vi "play_AFMss_integral_trajTrack_nod.vi"() -> ()   [LabVIEW 2017]
uses:
  controls/controlParams_tracktraj.ctl
  <vilib>/userdefined/High Color/nirio_resource_hc.ctl
  <vilib>/Utility/file.llb/Read From Spreadsheet File (DBL).vi
  <vilib>/FPGAPlugInAG/cRIO-9082/niLvFpga_Open_cRIO-9082.vi
  <vilib>/rvi/interface/common/dynamic/niFpgaDynamicAddResources.vi
  <vilib>/FPGAPlugInAG/Dynamic/niLvFpga_Reset_Dynamic.vi
  <vilib>/rvi/interface/common/niFpgaWaitOnOcc.vi
  <vilib>/Utility/error.llb/Error Cluster From Error Code.vi
  <vilib>/rvi/errors/niLvFpgaAdjustHostInterfaceError.vi
  <vilib>/FPGAPlugInAG/Dynamic/niLvFpga_Run_Dynamic.vi
  <vilib>/Utility/file.llb/Write To Spreadsheet File (DBL).vi
  <vilib>/FPGAPlugInAG/Dynamic/niLvFpga_Close_Dynamic.vi
  <vilib>/rvi/interface/nirviOpenFPGA/nirviOpenFPGA.xnode
  FPGA Bitfiles/XYpeizocontrol_FPGATargetSPARTA_AFMsscontroltraj_COTITsTKvb4.lvbitx
  <vilib>/rvi/interface/nirviMethod/nirviMethod.xnode
  <vilib>/rvi/interface/nirviReadWriteControl/nirviReadWriteControl.xnode
  <vilib>/rvi/interface/nirviCloseFPGA/nirviCloseFPGA.xnode
  <vilib>/FPGAPlugInAG/Dynamic/niLvFpga_ConfigureFifo_Dynamic.vi
  <vilib>/rvi/errors/niLvFpgaMergeErrorWithErrorCode.vi
  <vilib>/rvi/interface/Simulation/niFpgaSimulationCallBeginRW.vi
  <vilib>/FPGAPlugInAG/Dynamic/niLvFpga_ReadFifo_Dynamic.vi
  <vilib>/FPGAPlugInAG/Dynamic/niLvFpga_WriteFifo_Dynamic.vi
  NiFpgaLv.dll
panel:
  out "output array":dbl[][](array[numeric])
  in  "control_data_path":path=path "Z:/mpc-journal/step-exps/exp01Controls.csv"
  out "Actual Depth":u32
  out "YK TO":bool
  out "UK TO":bool
  out "yk":sgl
  out "loop ticks benchmark":sgl
  in  "Cluster":T1={"umax"=3.0, "y_ref(k)"=0.0, "Ki"=0.0, "y(k) (from plant)"=0.0, "ND"=0, "NS"=0, "u_Kx_ref(k)"=0.0} {"u_Kx_ref(k)" format="%#_13g"; "Ki" format="%#_13g"; "y_ref(k)" format="%#_13g"; "umax" format="%#_13g"}
  out "Unstable Traj":bool
  out "Control Loop Done":bool
  out "Elements Remaining":u32
  out "elements left":i32=1
  in  "reference traj path":path=path "Z:/mpc-journal/step-exps/ref_traj_track.csv"
  in  "outputData BOTH":path=path "Z:/mpc-journal/step-exps/exp01outputBOTH.csv"
  out "x+1":i32
  out "ND":i32
  out "NS":i32
  in  "Tab Control":enum32{"Custom Params", "Loaded Params"}(tab)
  in  "Nbar":dbl=1.253469179440319 format="%#_13g"
  in  "Ki":dbl=0.125346917944 format="%#_13g"
  out "Nbar":dbl=1.253469179440319 format="%#_13g"
  out "Ki":dbl=0.125346917944 format="%#_13g"
  out "ref":dbl format="%#_13g"
  in  "SettleTicks":i32=10
  in  "Stop":bool=TRUE
  out "y iter":i32
  out "u iter":i32
  out "size(s) 5":i32
  out "size(s)":i32
  out "K_in 2":sgl[](array[numeric])=[-0.023819132, 0.00010408472, 0.0, 0.0, 0.0, 0.0, 0.0, 0.0, 0.0]
  out "K_in":sgl[](array[numeric])=[-0.023819132, 0.00010408472, 0.0, 0.0, 0.0, 0.0, 0.0, 0.0, 0.0]
  out "C_in":sgl[](array[numeric])=[-8.076578e-08, -5.6617e-09, 2.3556278e-05, -6.9169624e-07, -0.005420799, 0.00037984832, -0.012524399, 0.0, 0.0]
  out "L_in":sgl[](array[numeric])=[-2254.4756, -17288.861, -3886.0125, -24956.67, -705.887, -3987.6506, -7.2153935, 0.0, 0.0] format="%#_11g"
  out "Bz_in":sgl[](array[numeric])=[-0.0016434871, -0.020676594, -0.010679029, -0.20639984, -0.030792456, -1.3413852, -0.02736353, 0.0, 0.0]
  in  "Iters":i32=25
  in  "Cont Run (F)":bool=TRUE
  in  "ymax":dbl=4.0 format="%#_13g"
  in  "umax":dbl=1.0 format="%#_13g"
  in  "TsTicks":i32=1600
  # "Manually define Parameters"
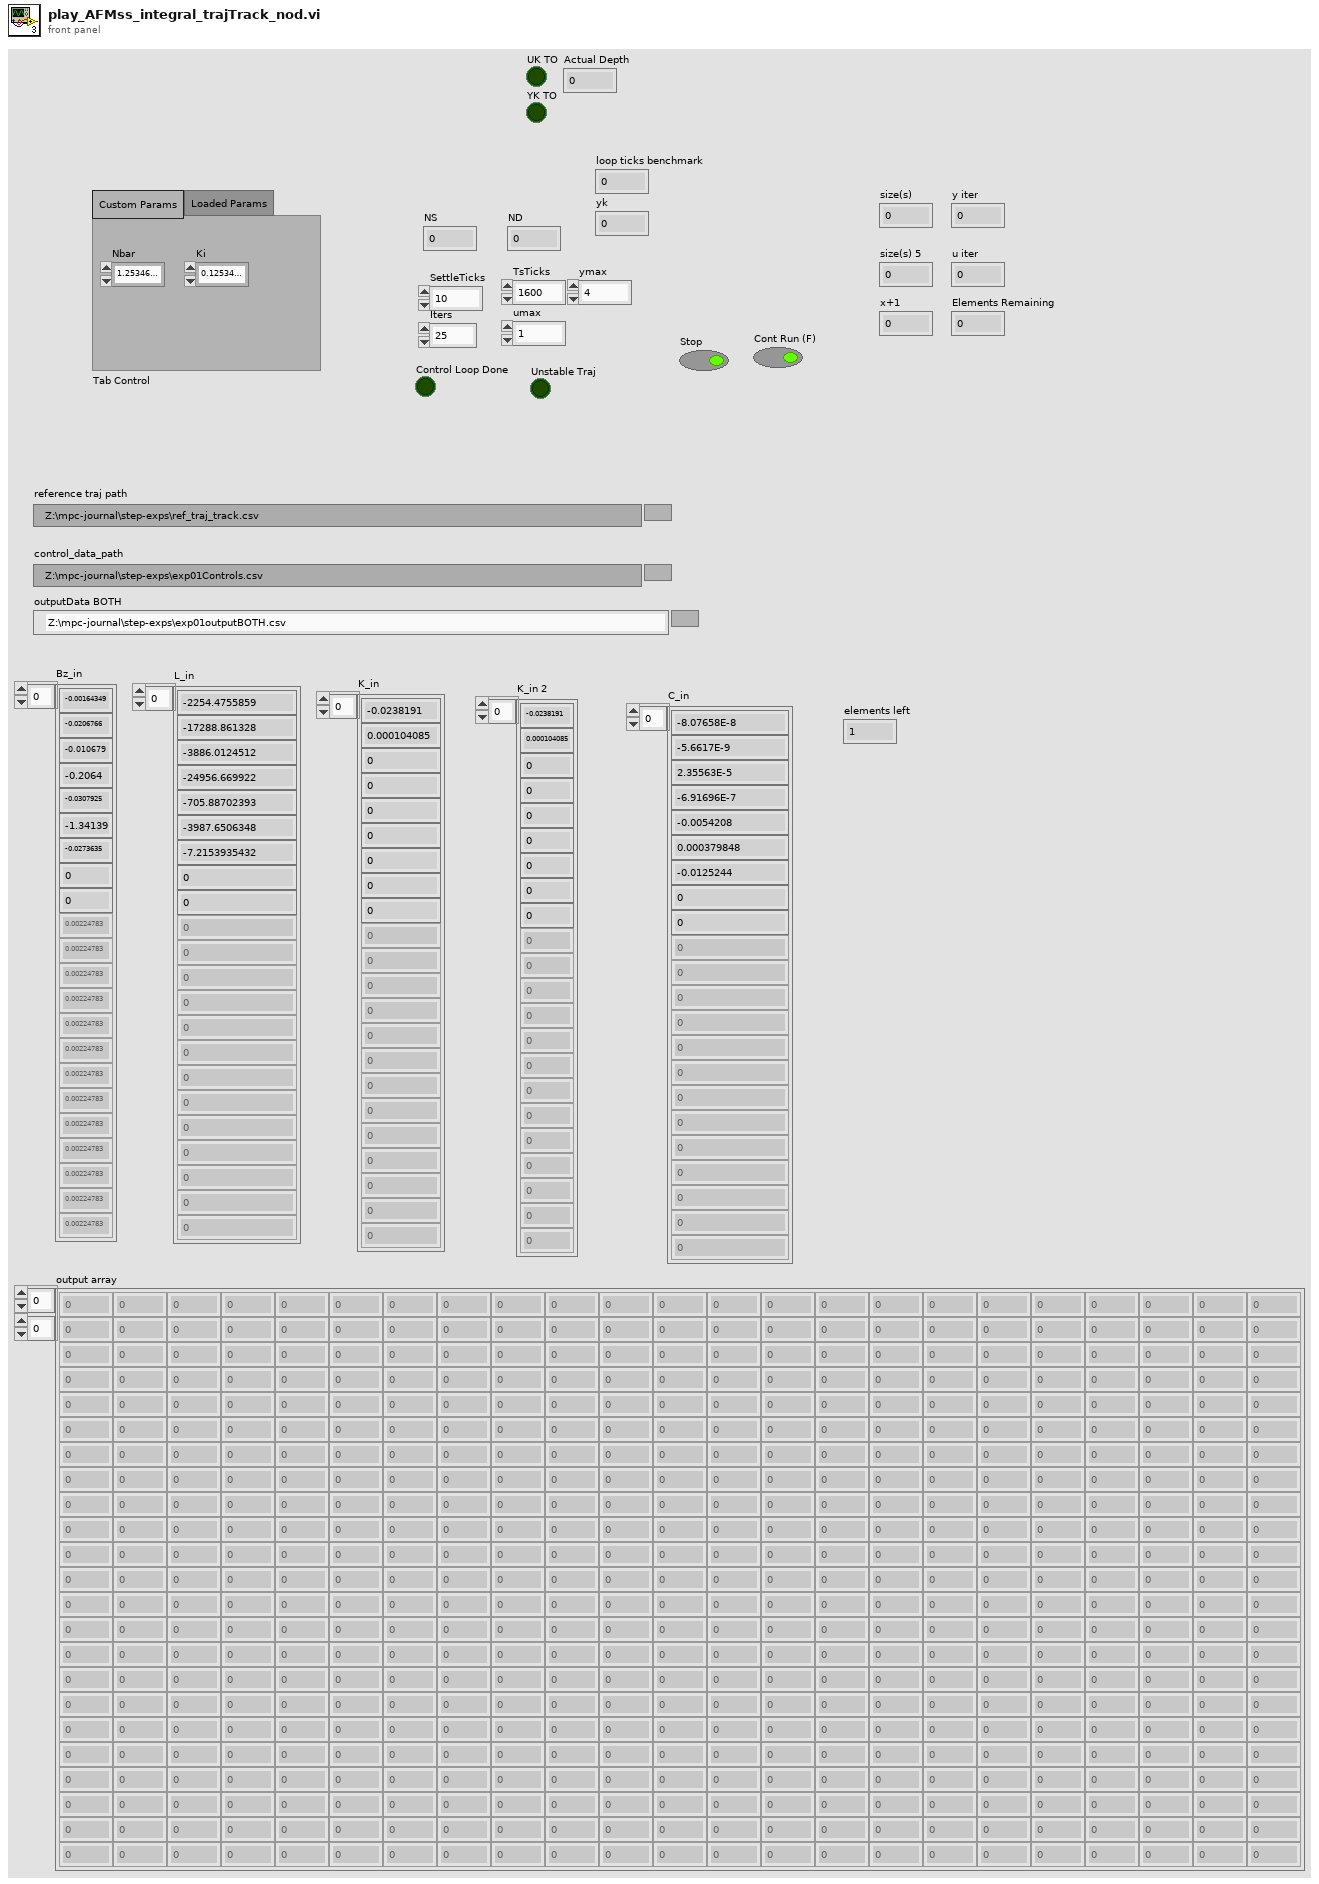
[diagram p1: front panel]
types:
  T1 = typedef "controlParams_tracktraj.ctl" = cluster{"umax":sgl, "y_ref(k)":sgl, "Ki":sgl, "y(k) (from plant)":sgl, "ND":i16, "NS":i16, "u_Kx_ref(k)":sgl}
  T2 = typedef "nirio_resource_hc.ctl" = tag
  T3 = typedef "ControlParams.ctl" = cluster{"NS":i32, "ND":i32, "Nbar":dbl, "Ki":dbl, "ref":dbl}
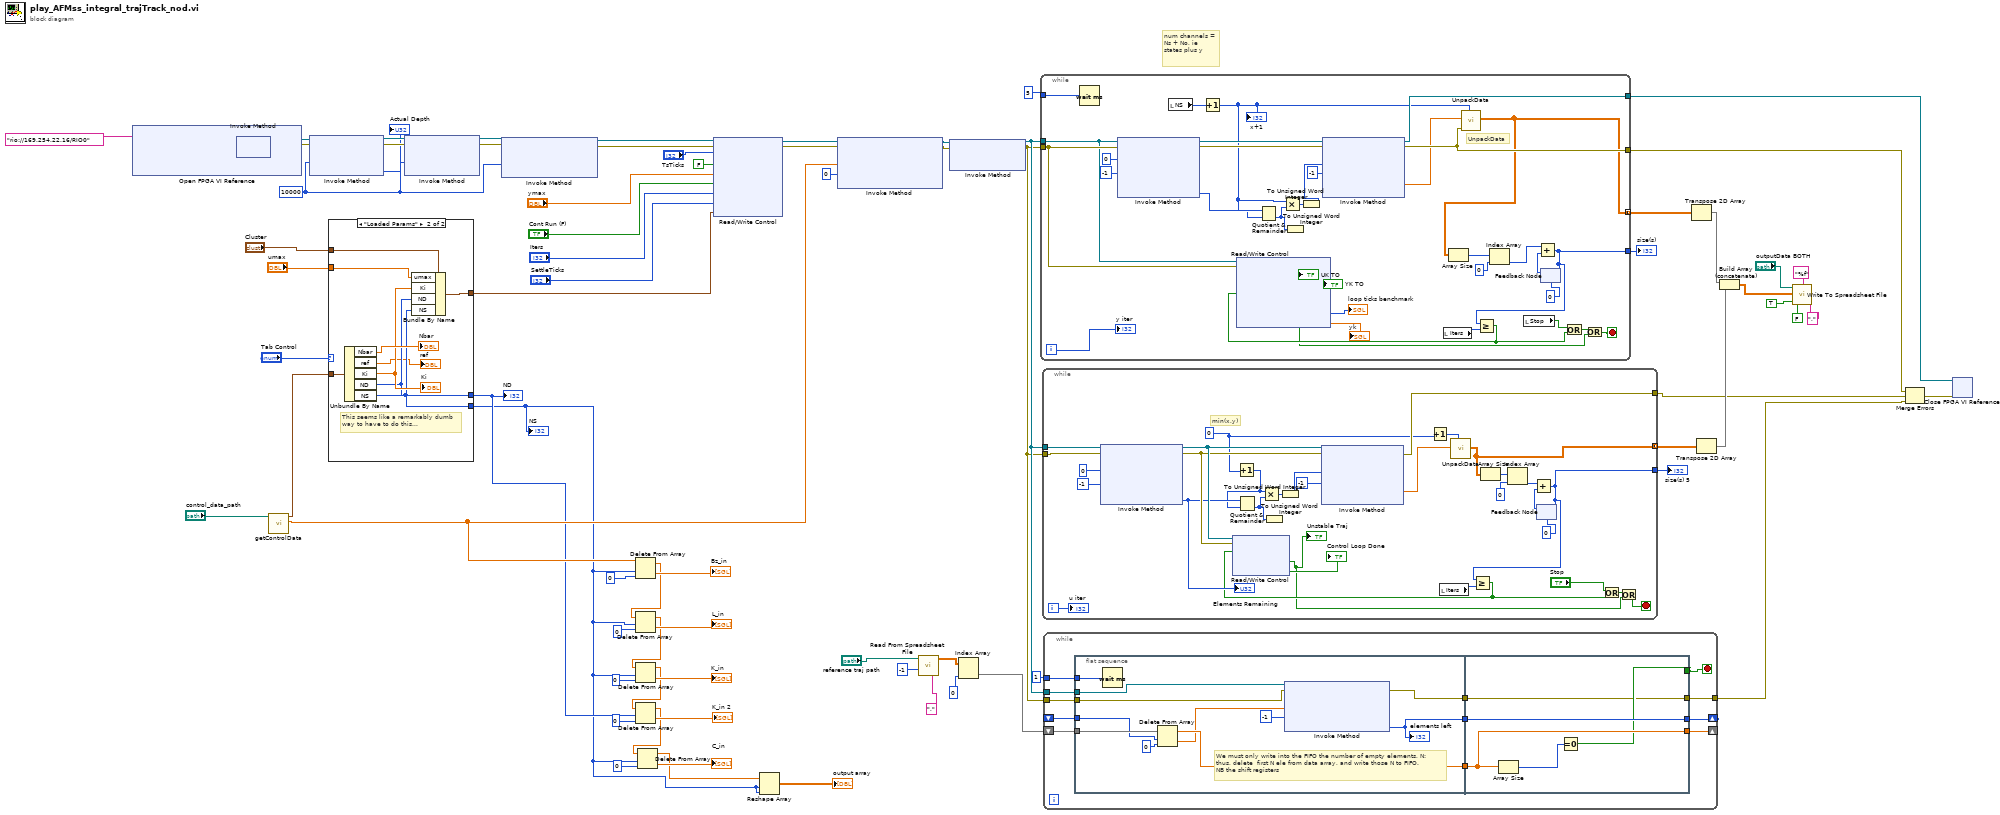
[diagram p0: block diagram]
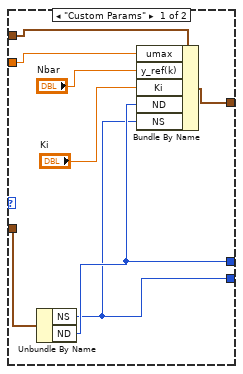
[diagram p2: hidden frame]
diagram:
  w38 = 10000
  # "num channels = Ns + No, ie states plus y"
  n1 = xnode "Open FPGA VI Reference"("resource name"=T2 "rio://169.254.22.16/RIO0") -> ("FPGA VI Reference Out"=w33:refnum<k20>, "error out"=w32:errorcluster)  [unwired: 1 in]
  n2 = xnode "Invoke Method"("FPGA VI Reference In"=w33, "error in"=w32) -> ("FPGA VI Reference Out"=w45:refnum<k20>, "error out"=w44:errorcluster)
  n3 = call "getControlData.vi"("system matricec path"="control_data_path") -> ("AllMatrix"=w37:dbl[], "controlParams"=w36:T3)  [unwired: 9 in]
  n4 = xnode "Invoke Method"("FPGA VI Reference In"=w45, "error in"=w44, "Requested Depth"=w38) -> ("FPGA VI Reference Out"=w76:refnum<k20>, "error out"=w75:errorcluster, "Actual Depth"=→"Actual Depth":u32)
  n5 = case shown="\"Loaded Params\"" "Tab Control" {
    tunnel: w36 -> [w84 w93]
    tunnel: [w78 w88] -> w2
    tunnel: [w79 w89] -> w34
    tunnel: "umax" -> [w83 w86]
    tunnel: [w81 w90] -> w10
    tunnel: "Cluster" -> [w77 w87]
    frame "Custom Params" {
      n6 = Unbundle By Name(w84) -> ("NS"=w78:i32, "ND"=w79:i32)
      n7 = Bundle By Name(cluster=w77, "umax"=w83, "y_ref(k)"="Nbar", "Ki"="Ki", "ND"=w79, "NS"=w78) -> (w81:T1)
    }
    frame "Loaded Params" {
      # "This seems like a remarkably dumb\nway to have to do this..."
      n8 = Unbundle By Name(w93) -> ("Nbar"=→"Nbar":dbl, "ref"=→"ref":dbl, "Ki"=w91:dbl, "ND"=w89:i32, "NS"=w88:i32)
      "Ki" <- w91
      n9 = Bundle By Name(cluster=w87, "umax"=w86, "Ki"=w91, "ND"=w89, "NS"=w88) -> (w90:T1)
    }
  }
  "NS" <- w2
  "ND" <- w34
  n10 = xnode "Invoke Method"("FPGA VI Reference In"=w76, "error in"=w75, "Requested Depth"=w38) -> ("FPGA VI Reference Out"=w42:refnum<k20>, "error out"=w41:errorcluster)  [unwired: 1 out]
  n11 = xnode "Invoke Method"("FPGA VI Reference In"=w42, "error in"=w41, "Requested Depth"=w38) -> ("FPGA VI Reference Out"=w40:refnum<k20>, "error out"=w39:errorcluster)  [unwired: 1 out]
  n12 = Delete From Array(array=w37, length=w2, index=0) -> (deleted portion=→"Bz_in":dbl[], array with subset deleted=w60:dbl[])
  n13 = Delete From Array(array=w60, length=w2, index=0) -> (deleted portion=→"L_in":dbl[], array with subset deleted=w57:dbl[])
  n14 = Delete From Array(array=w57, length=w2, index=0) -> (deleted portion=→"K_in":dbl[], array with subset deleted=w53:dbl[])
  n15 = Delete From Array(array=w53, length=w34, index=0) -> (deleted portion=→"K_in 2":dbl[], array with subset deleted=w50:dbl[])
  n16 = Delete From Array(array=w50, length=w2, index=0) -> (deleted portion=→"C_in":dbl[], array with subset deleted=w3:dbl[])
  n17 = xnode "Read/Write Control"("FPGA VI Reference In"=w40, "error in"=w39, "TsTicks"="TsTicks", "Abort"=FALSE, "ymax"="ymax", "False  = cont run"="Cont Run (F)", "iters"="Iters", "Settle Ticks"="SettleTicks", "Cluster"=w10) -> ("FPGA VI Reference Out"=w65:refnum<k20>, "error out"=w64:errorcluster)
  n18 = Reshape Array(w3, w2, w2) -> (→"output array":dbl[][])
  n19 = xnode "Invoke Method"("FPGA VI Reference In"=w65, "error in"=w64, "Data"=w37, "Timeout (ms)"=0) -> ("FPGA VI Reference Out"=w68:refnum<k20>, "error out"=w67:errorcluster)  [unwired: 1 out]
  n20 = call-poly <vilib>:"Read From Spreadsheet File.vi"("delimiter (\\t)"=",", "number of rows (all:-1)"=-1, "file path (dialog if empty)"="reference traj path") -> ("all rows"=w17:dbl[][])  [unwired: 4 in, 4 out]
  n21 = xnode "Invoke Method"("FPGA VI Reference In"=w68, "error in"=w67) -> ("FPGA VI Reference Out"=w8:refnum<k20>, "error out"=w7:errorcluster)  [unwired: 1 in]
  n22 = Index Array(array=w17, index (col)=0 ("dimension size")) -> (element=w15:dbl[])  [unwired: 1 in]
  n23 = while {
    tunnel: 5 -> [w128]
    tunnel: w8 -> [w106]
    tunnel: w7 -> [w107]
    tunnel: [w120] -> w14
    tunnel: [w119] -> w63
    tunnel: [w105] -> w48 mode=concatenating
    tunnel: [w103] -> w46
    i -> [w104]
    stop <- w98 stop-if-true
    # "UnpackData"
    n24 = Wait (ms)(milliseconds to wait=w128) -> ()  [unwired: 1 out]
    n25 = xnode "Invoke Method"("FPGA VI Reference In"=w106, "error in"=w107, "Number of Elements"=0 ("Timeout (ms)"), "Timeout (ms)"=-1) -> ("FPGA VI Reference Out"=w124:refnum<k20>, "error out"=w125:errorcluster, "Elements Remaining"=w115:u32)  [unwired: 1 out]
    n26 = local read "NS"() -> (w114:i32)
    n27 = Increment(x=w114) -> (x+1=w113:i32)
    "x+1" <- w113
    n28 = Quotient & Remainder(x=w115, y=w113) -> (floor(x/y)=w117:u32)  [unwired: 1 out]
    n29 = Multiply(x=w113, y=w117) -> (x*y=w122:u32)
    n30 = To Unsigned Word Integer(number=w117) -> ()  [unwired: 1 out]
    n31 = To Unsigned Word Integer(number=w122) -> (unsigned 16bit integer=w118:u16)
    n32 = xnode "Invoke Method"("FPGA VI Reference In"=w124, "error in"=w125, "Number of Elements"=w118, "Timeout (ms)"=-1) -> ("FPGA VI Reference Out"=w119:refnum<k20>, "error out"=w120:errorcluster, "Data"=w112:sgl[])  [unwired: 1 out]
    n33 = local read "Iters"() -> (w116:i32)
    n34 = call "UnpackData.vi"("NumChannels"=w113, "error In"=w120, "1D Data In"=w112) -> ("2D Data Out"=w105:dbl[][])  [unwired: 7 in, 1 out]
    n35 = Array Size(array=w105) -> (size(s)=w111:i32[])
    n36 = Index Array(array=w111, index=0) -> (element=w109:i32)
    n37 = local read "Stop"() -> (w101:bool)
    n38 = feedback #1(0) -> (w110:i32)
    n39 = Add(x=w109, y=w110) -> (x+y=w103:i32)
    n40 = Greater Or Equal?(x=w103, y=w116) -> (x >= y?=w102:bool)
    n41 = xnode "Read/Write Control"("FPGA VI Reference In"=w106, "error in"=w107, "Abort"=w102) -> ("UK TO"=→"UK TO":bool, "YK TO"=→"YK TO":bool, "Unstable Traj"=w99:bool, "Loop Ticks (benchmark)"=→"loop ticks benchmark":i16, "yk"=→"yk":sgl)  [unwired: 2 out]
    n42 = feedback-in #1(w103) -> ()
    n43 = Or(x=w101, y=w102) -> (x .or. y?=w100:bool)
    n44 = Or(x=w100, y=w99) -> (x .or. y?=w98:bool)
    "y iter" <- w104
  }
  "size(s)" <- w46
  n45 = while {
    tunnel: [w138] -> w35 mode=concatenating
    tunnel: w8 -> [w146]
    tunnel: w7 -> [w145]
    tunnel: [w143] -> w47
    tunnel: [w134] -> w12
    i -> [w144]
    stop <- w133 stop-if-true
    w129 = i16 0 ("x")
    # "min(x,y)"
    n46 = xnode "Invoke Method"("FPGA VI Reference In"=w146, "error in"=w145, "Number of Elements"=0 ("Timeout (ms)"), "Timeout (ms)"=-1) -> ("FPGA VI Reference Out"=w154:refnum<k20>, "error out"=w153:errorcluster, "Elements Remaining"=w150:u32)  [unwired: 1 out]
    "Elements Remaining" <- w150
    n47 = Increment(x=w129) -> (x+1=w148:i16)
    n48 = Quotient & Remainder(x=w150, y=w148) -> (floor(x/y)=w151:u32)  [unwired: 1 out]
    n49 = Multiply(x=w148, y=w151) -> (x*y=w152:u32)
    n50 = To Unsigned Word Integer(number=w151) -> ()  [unwired: 1 out]
    n51 = To Unsigned Word Integer(number=w152) -> (unsigned 16bit integer=w149:u16)
    n52 = xnode "Invoke Method"("FPGA VI Reference In"=w154, "error in"=w153, "Number of Elements"=w149, "Timeout (ms)"=-1) -> ("error out"=w134:errorcluster, "Data"=w140:sgl[])  [unwired: 2 out]
    n53 = Increment(x=w129) -> (x+1=w137:i16)
    n54 = local read "Iters"() -> (w155:i32)
    n55 = call "UnpackData.vi"("NumChannels"=w137, "1D Data In"=w140) -> ("2D Data Out"=w138:dbl[][])  [unwired: 8 in, 1 out]
    n56 = Array Size(array=w138) -> (size(s)=w135:i32[])
    n57 = Index Array(array=w135, index=0) -> (element=w139:i32)
    n58 = feedback #2(0) -> (w147:i32)
    n59 = Add(x=w139, y=w147) -> (x+y=w143:i32)
    n60 = Greater Or Equal?(x=w143, y=w155) -> (x >= y?=w142:bool)
    n61 = xnode "Read/Write Control"("FPGA VI Reference In"=w154, "error in"=w153, "Abort"=w142) -> ("Unstable Traj"=w130:bool, "Loop Done"=→"Control Loop Done":bool)  [unwired: 2 out]
    "Unstable Traj" <- w130
    n62 = feedback-in #2(w143) -> ()
    n63 = Or(x="Stop", y=w142) -> (x .or. y?=w132:bool)
    n64 = Or(x=w132, y=w130) -> (x .or. y?=w133:bool)
    "u iter" <- w144
  }
  "size(s) 5" <- w47
  n65 = while {
    tunnel: [w169] -> w11
    tunnel: 1 -> [w171]
    shift-right: [w164] -> _
    shift-left: _ -> [w168]
    shift-right: [w162] -> _
    shift-left: w15 -> [w170]
    tunnel: w8 -> [w161]
    tunnel: w7 -> [w160]
    stop <- w165 stop-if-true
    n66 = flat-sequence {
      tunnel: w171 -> [w182]
      tunnel: w170 -> [w177]
      tunnel: w168 -> [w173]
      tunnel: [w180] -> w167
      tunnel: [w178] -> w166
      tunnel: [w179] -> w163
      tunnel: w161 -> [w175]
      tunnel: w160 -> [w174]
      tunnel: [w187] -> w164
      tunnel: [w183] -> w169
      tunnel: w167 -> [w183]
      tunnel: w166 -> [w187]
      tunnel: [w184] -> w165
      tunnel: w163 -> [w185]
      tunnel: [w185] -> w162
      frame #0 {
        # "We must only write into the FIFO the number of empty elements, N:\nthus, delete  first N ele from data array, and write those N to FIFO.\nNB the shift registers"
        n67 = Wait (ms)(milliseconds to wait=w182) -> ()  [unwired: 1 out]
        n68 = Delete From Array(array=w177, length=w173, index=0) -> (deleted portion=w176:dbl[], array with subset deleted=w179:dbl[])
        n69 = xnode "Invoke Method"("FPGA VI Reference In"=w175, "error in"=w174, "Data"=w176, "Timeout (ms)"=-1) -> ("error out"=w180:errorcluster, "Empty Elements Remaining"=w178:u32)  [unwired: 1 out]
        "elements left" <- w178
      }
      frame #1 {
        n70 = Array Size(array=w185) -> (size(s)=w186:i32)
        n71 = Equal To 0?(x=w186) -> (x = 0?=w184:bool)
      }
    }
  }
  n72 = Transpose 2D Array(2D array=w48) -> (transposed array=w29:dbl[][])
  n73 = Transpose 2D Array(2D array=w35) -> (transposed array=w28:dbl[][])
  n74 = Build Array (concatenate)(w29, w28) -> (w22:dbl[][])
  n75 = call-poly <vilib>:"Write To Spreadsheet File.vi"("delimiter (\\t)"=",", "transpose? (no:F)"=TRUE, "format (%.3f)"="%f", "append to file? (new file:F)"=FALSE, "2D data"=w22, "file path (dialog if empty)"="outputData BOTH") -> ()  [unwired: 2 in, 1 out]
  n76 = Merge Errors(w14, w12, w11) -> (w13:errorcluster)
  n77 = xnode "Close FPGA VI Reference"("FPGA VI Reference In"=w63, "error in"=w13) -> ()  [unwired: 1 out]
